vi "Calculate FOV Range.vi"(9 "Center Voltage":dbl format="%#_13g", 10 "Galvo Step Stize (px/V)":dbl format="%#_13g", 11 "Num. Px(Half FOV)":u16) -> (0 "Amplitude":dbl, 1 "Galvo Step Stize (px/V) Out":dbl format="%#_13g", 2 "Stop Value":dbl, 3 "Start Value":dbl)   [LabVIEW 2018]
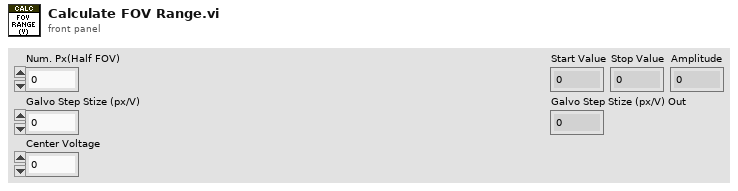
[diagram p1: front panel]
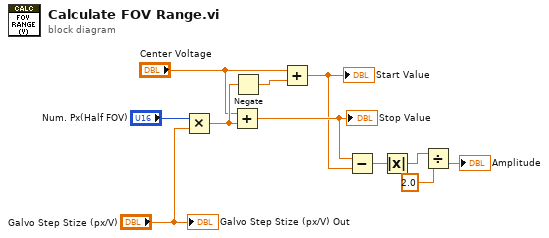
[diagram p0: block diagram]
diagram:
  n1 = Multiply(x="Num. Px(Half FOV)", y="Galvo Step Stize (px/V)") -> (x*y=w9:dbl)
  n2 = Add(x="Center Voltage", y=w9) -> (x+y=w6:dbl)
  "Stop Value" <- w6
  n3 = Negate(x=w9) -> (-x=w7:dbl)
  n4 = Add(x="Center Voltage", y=w7) -> (x+y=w5:dbl)
  "Start Value" <- w5
  n5 = Subtract(x=w6, y=w5) -> (x-y=w4:dbl)
  n6 = Absolute Value(x=w4) -> (abs(x)=w3:dbl)
  n7 = Divide(x=w3, y=2.0 ("x")) -> (x/y=→"Amplitude":dbl)
  "Galvo Step Stize (px/V) Out" <- "Galvo Step Stize (px/V)"
